vi "7seg.vi"() -> ()   [LabVIEW 2019]
panel:
  out "数値":i32
  out "文字列":string
  in  "スライド 4":i64(slide) scale=0.0..1.0
  in  "スライド 3":i64(slide) scale=0.0..1.0
  in  "スライド 2":i64(slide) scale=0.0..1.0
  in  "スライド":i64(slide) scale=0.0..1.0
  out "ブール 7":bool
  out "ブール 6":bool
  out "ブール 5":bool
  out "ブール 4":bool
  out "ブール 3":bool
  out "ブール 2":bool
  out "ブール":bool
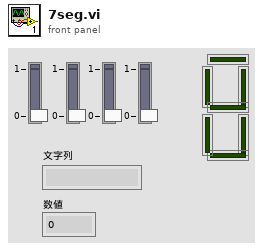
[diagram p1: front panel]
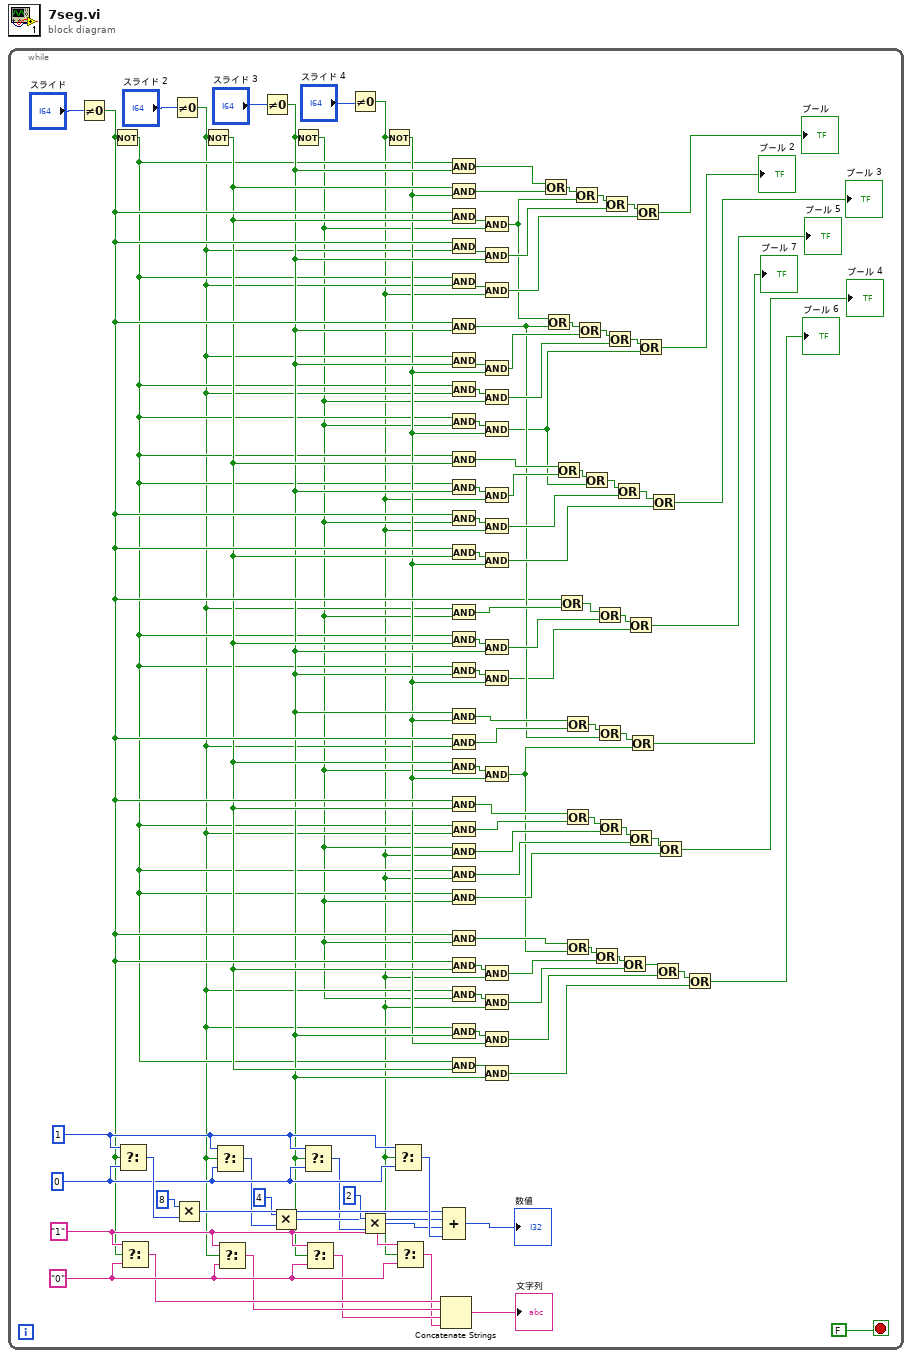
[diagram p0: block diagram]
diagram:
  n1 = while {
    stop <- FALSE stop-if-true
    w61 = 1
    w62 = 0
    w100 = "1"
    w99 = "0"
    n2 = Not Equal To 0?(x="スライド") -> (x != 0?=w26:bool)
    n3 = Not(x=w26) -> (.not. x?=w13:bool)
    n4 = Select(t=w61, s=w26, f=w62) -> (s? t:f=w63:i32)
    n5 = Select(t=w100, s=w26, f=w99) -> (s? t:f=w98:string)
    n6 = Not Equal To 0?(x="スライド 2") -> (x != 0?=w7:bool)
    n7 = Multiply(x=8, y=w63) -> (x*y=w58:i32)
    n8 = Not(x=w7) -> (.not. x?=w22:bool)
    n9 = Select(t=w61, s=w7, f=w62) -> (s? t:f=w53:i32)
    n10 = Select(t=w100, s=w7, f=w99) -> (s? t:f=w97:string)
    n11 = Not Equal To 0?(x="スライド 3") -> (x != 0?=w21:bool)
    n12 = Multiply(x=4, y=w53) -> (x*y=w54:i32)
    n13 = Not(x=w21) -> (.not. x?=w6:bool)
    n14 = Select(t=w61, s=w21, f=w62) -> (s? t:f=w51:i32)
    n15 = Select(t=w100, s=w21, f=w99) -> (s? t:f=w96:string)
    n16 = Not Equal To 0?(x="スライド 4") -> (x != 0?=w5:bool)
    n17 = Multiply(x=2, y=w51) -> (x*y=w52:i32)
    n18 = Not(x=w5) -> (.not. x?=w15:bool)
    n19 = Select(t=w61, s=w5, f=w62) -> (s? t:f=w60:i32)
    n20 = Select(t=w100, s=w5, f=w99) -> (s? t:f=w95:string)
    n21 = Concatenate Strings(w98, w97, w96, w95) -> (→"文字列":string)
    n22 = Compound Arithmetic op=ADD(w58, w54, w52, w60) -> (→"数値":i32)
    n23 = And(x=w13, y=w21) -> (x .and. y?=w32:bool)
    n24 = And(x=w22, y=w15) -> (x .and. y?=w91:bool)
    n25 = And(x=w26, y=w22) -> (x .and. y?=w93:bool)
    n26 = And(x=w26, y=w7) -> (x .and. y?=w92:bool)
    n27 = And(x=w13, y=w7) -> (x .and. y?=w88:bool)
    n28 = And(x=w26, y=w21) -> (x .and. y?=w36:bool)
    n29 = And(x=w7, y=w21) -> (x .and. y?=w83:bool)
    n30 = And(x=w13, y=w7) -> (x .and. y?=w82:bool)
    n31 = And(x=w13, y=w6) -> (x .and. y?=w81:bool)
    n32 = And(x=w13, y=w22) -> (x .and. y?=w40:bool)
    n33 = And(x=w13, y=w21) -> (x .and. y?=w73:bool)
    n34 = And(x=w26, y=w6) -> (x .and. y?=w72:bool)
    n35 = And(x=w26, y=w22) -> (x .and. y?=w71:bool)
    n36 = And(x=w7, y=w6) -> (x .and. y?=w49:bool)
    n37 = And(x=w13, y=w22) -> (x .and. y?=w48:bool)
    n38 = And(x=w13, y=w21) -> (x .and. y?=w47:bool)
    n39 = And(x=w21, y=w15) -> (x .and. y?=w43:bool)
    n40 = And(x=w26, y=w7) -> (x .and. y?=w42:bool)
    n41 = And(x=w22, y=w6) -> (x .and. y?=w39:bool)
    n42 = And(x=w26, y=w22) -> (x .and. y?=w35:bool)
    n43 = And(x=w13, y=w7) -> (x .and. y?=w34:bool)
    n44 = And(x=w6, y=w5) -> (x .and. y?=w14:bool)
    n45 = And(x=w13, y=w5) -> (x .and. y?=w12:bool)
    n46 = And(x=w13, y=w6) -> (x .and. y?=w11:bool)
    n47 = And(x=w26, y=w6) -> (x .and. y?=w28:bool)
    n48 = And(x=w26, y=w22) -> (x .and. y?=w2:bool)
    n49 = And(x=w7, y=w6) -> (x .and. y?=w1:bool)
    n50 = And(x=w7, y=w21) -> (x .and. y?=w3:bool)
    n51 = And(x=w13, y=w22) -> (x .and. y?=w20:bool)
    n52 = And(x=w93, y=w6) -> (x .and. y?=w77:bool)
    n53 = And(x=w92, y=w21) -> (x .and. y?=w87:bool)
    n54 = And(x=w88, y=w5) -> (x .and. y?=w85:bool)
    n55 = And(x=w83, y=w15) -> (x .and. y?=w76:bool)
    n56 = And(x=w82, y=w6) -> (x .and. y?=w75:bool)
    n57 = And(x=w81, y=w15) -> (x .and. y?=w29:bool)
    n58 = And(x=w73, y=w5) -> (x .and. y?=w70:bool)
    n59 = And(x=w72, y=w5) -> (x .and. y?=w67:bool)
    n60 = And(x=w71, y=w15) -> (x .and. y?=w65:bool)
    n61 = And(x=w48, y=w21) -> (x .and. y?=w45:bool)
    n62 = And(x=w47, y=w15) -> (x .and. y?=w27:bool)
    n63 = And(x=w39, y=w15) -> (x .and. y?=w8:bool)
    n64 = And(x=w2, y=w5) -> (x .and. y?=w23:bool)
    n65 = And(x=w1, y=w5) -> (x .and. y?=w4:bool)
    n66 = And(x=w3, y=w15) -> (x .and. y?=w9:bool)
    n67 = And(x=w20, y=w21) -> (x .and. y?=w17:bool)
    n68 = Or(x=w32, y=w91) -> (x .or. y?=w90:bool)
    n69 = Or(x=w77, y=w36) -> (x .or. y?=w78:bool)
    n70 = Or(x=w40, y=w70) -> (x .or. y?=w69:bool)
    n71 = Or(x=w26, y=w49) -> (x .or. y?=w50:bool)
    n72 = Or(x=w43, y=w42) -> (x .or. y?=w41:bool)
    n73 = Or(x=w35, y=w34) -> (x .or. y?=w33:bool)
    n74 = Or(x=w28, y=w8) -> (x .or. y?=w25:bool)
    n75 = Or(x=w90, y=w77) -> (x .or. y?=w89:bool)
    n76 = Or(x=w78, y=w76) -> (x .or. y?=w79:bool)
    n77 = Or(x=w69, y=w29) -> (x .or. y?=w68:bool)
    n78 = Or(x=w25, y=w23) -> (x .or. y?=w24:bool)
    n79 = Or(x=w50, y=w45) -> (x .or. y?=w46:bool)
    n80 = Or(x=w41, y=w36) -> (x .or. y?=w38:bool)
    n81 = Or(x=w33, y=w14) -> (x .or. y?=w31:bool)
    n82 = Or(x=w89, y=w87) -> (x .or. y?=w86:bool)
    n83 = Or(x=w79, y=w75) -> (x .or. y?=w80:bool)
    n84 = Or(x=w68, y=w67) -> (x .or. y?=w66:bool)
    n85 = Or(x=w24, y=w4) -> (x .or. y?=w19:bool)
    n86 = Or(x=w46, y=w27) -> (x .or. y?=→"ブール 5":bool)
    n87 = Or(x=w31, y=w12) -> (x .or. y?=w30:bool)
    n88 = Or(x=w38, y=w8) -> (x .or. y?=→"ブール 7":bool)
    n89 = Or(x=w86, y=w85) -> (x .or. y?=→"ブール":bool)
    n90 = Or(x=w80, y=w29) -> (x .or. y?=→"ブール 2":bool)
    n91 = Or(x=w66, y=w65) -> (x .or. y?=→"ブール 3":bool)
    n92 = Or(x=w19, y=w9) -> (x .or. y?=w18:bool)
    n93 = Or(x=w30, y=w11) -> (x .or. y?=→"ブール 4":bool)
    n94 = Or(x=w18, y=w17) -> (x .or. y?=→"ブール 6":bool)
  }
